vi "CONVERT HEX TO CURRENT.vi"(11 "HEX STRING":string) -> (2 "CURRENT":dbl[unit])   [LabVIEW 2018]
uses:
  <vilib>/Utility/error.llb/whitespace.ctl
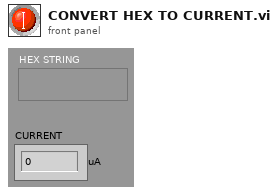
[diagram p1: front panel]
types:
  T1 = typedef "whitespace.ctl" = u16
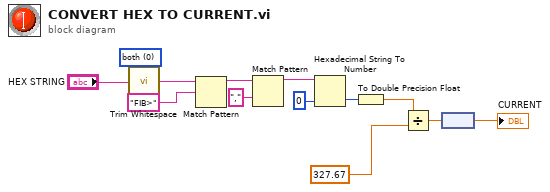
[diagram p0: block diagram]
diagram:
  w13 = T1 0 items=["both", "start of string", "end of string"] ("location (both)")
  n1 = call <vilib>:"Trim Whitespace.vi"("string"="HEX STRING", "location (both)"=w13) -> ("trimmed string"=w12:string)
  n2 = Match Pattern(string=w12, regular expression="FIB>") -> (before substring=w10:string)  [unwired: 1 in, 3 out]
  n3 = Match Pattern(string=w10, regular expression=",") -> (before substring=w7:string)  [unwired: 1 in, 3 out]
  n4 = Hexadecimal String To Number(string=w7, default (0uL)=i16 0 ("default (0 U32)")) -> (number=w1:i16)  [unwired: 1 in, 1 out]
  n5 = To Double Precision Float(number=w1) -> (double precision float=w4:dbl)
  n6 = Divide(x=w4, y=327.67) -> (x/y=w3:dbl)
  n7 = node(w3) -> (→"CURRENT":dbl[unit])
